vi "HEARTBEAT.vi"(0 "Custom Mode":u32, 5 "type":u8=6, 7 "autopilot":u8=8, 9 "base_mode":u8, 11 "system_status":u8) -> (4 "MAVLink Message":u8[](array[numeric]))   [LabVIEW 2014]
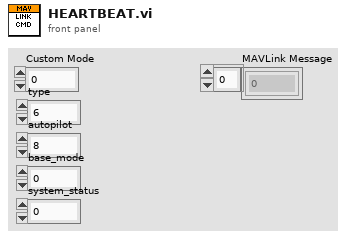
[diagram p1: front panel]
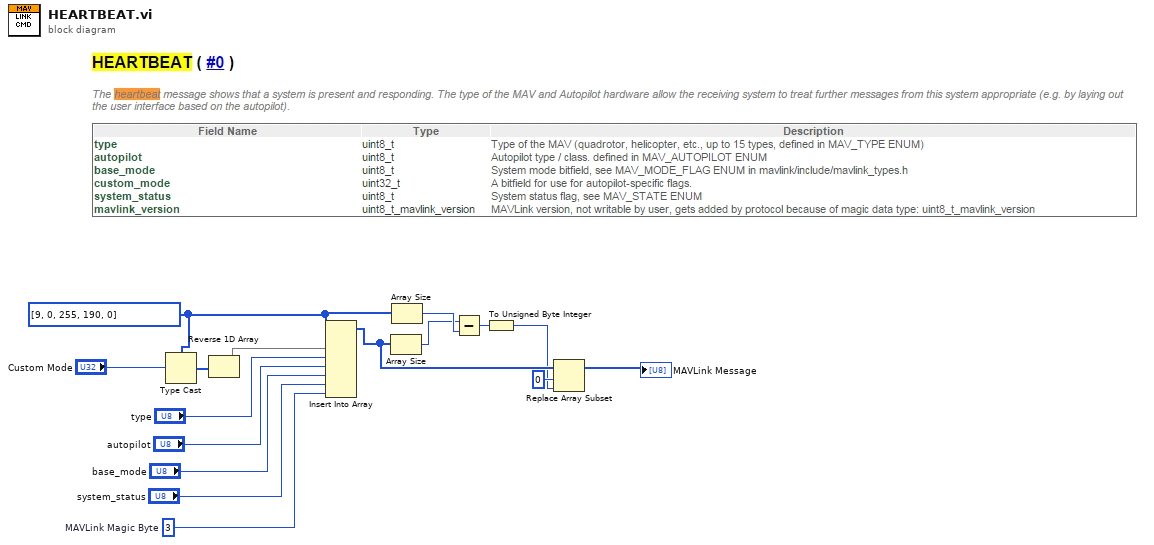
[diagram p0: block diagram]
diagram:
  w9 = u8 3  # MAVLink Magic Byte
  w8 = u8[] [9, 0, 255, 190, 0]
  n1 = Type Cast(type=w8, x="Custom Mode") -> (*(type *) &x=w15:u8[])
  n2 = Reverse 1D Array(array=w15) -> (reversed array=w14:u8[])
  n3 = Insert Into Array(array=w8, new element #1=w14, new element #2="type", new element #3="autopilot", new element #4="base_mode", new element #5="system_status", new element #6=w9) -> (w4:u8[])  [unwired: 1 in]
  n4 = Array Size(array=w4) -> (size(s)=w6:i32)
  n5 = Array Size(array=w8) -> (size(s)=w7:i32)
  n6 = Subtract(x=w6, y=w7) -> (x-y=w5:i32)
  n7 = To Unsigned Byte Integer(number=w5) -> (unsigned 8bit integer=w2:u8)
  n8 = Replace Array Subset(array=w4, new element=w2, index=0) -> (→"MAVLink Message":u8[])
